vi "Coherent FGV.vi"(7 "Funtion":T1(ring), 8 "error in":errorcluster, 9 "Power(mW)":dbl, 10 "Operating Mode":u16(ring) items=["CW Constant Power", "CW Constant Current", "Pulsed Digital", "Pulsed Analog", "Pulsed Mixed"], 11 "VISA resource name in":refnum<visa-resource-name>) -> (0 "error out":errorcluster, 3 "Laser State":T2)   [LabVIEW 2019, in "Coherent.lvlib"]
uses:
  Coherent.lvlib
  <vilib>/Instr/_visa.llb/VISA Configure Serial Port (Instr).vi
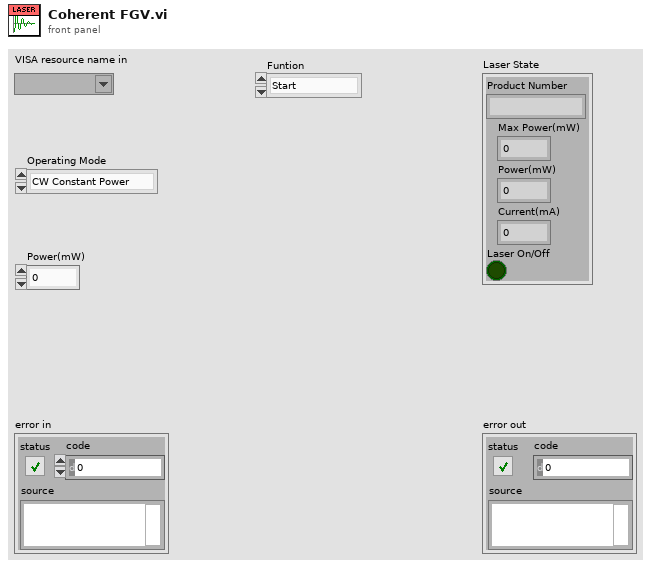
[diagram p1: front panel]
types:
  T1 = enum16{"Start", "Get State", "On", "Off", "Set Power", "Change Mode", "Close"}
  T2 = cluster{"Product Number":string, "Max Power(mW)":dbl, "Power(mW)":dbl, "Current(mA)":dbl, "Laser On/Off":bool}
  T3 = cluster{"Laser State":cluster{"Product Number":string, "Max Power(mW)":dbl, "Power(mW)":dbl, "Current(mA)":dbl, "Laser On/Off":bool}, "VISA resource name":refnum<visa-resource-name>, "Mode":string}
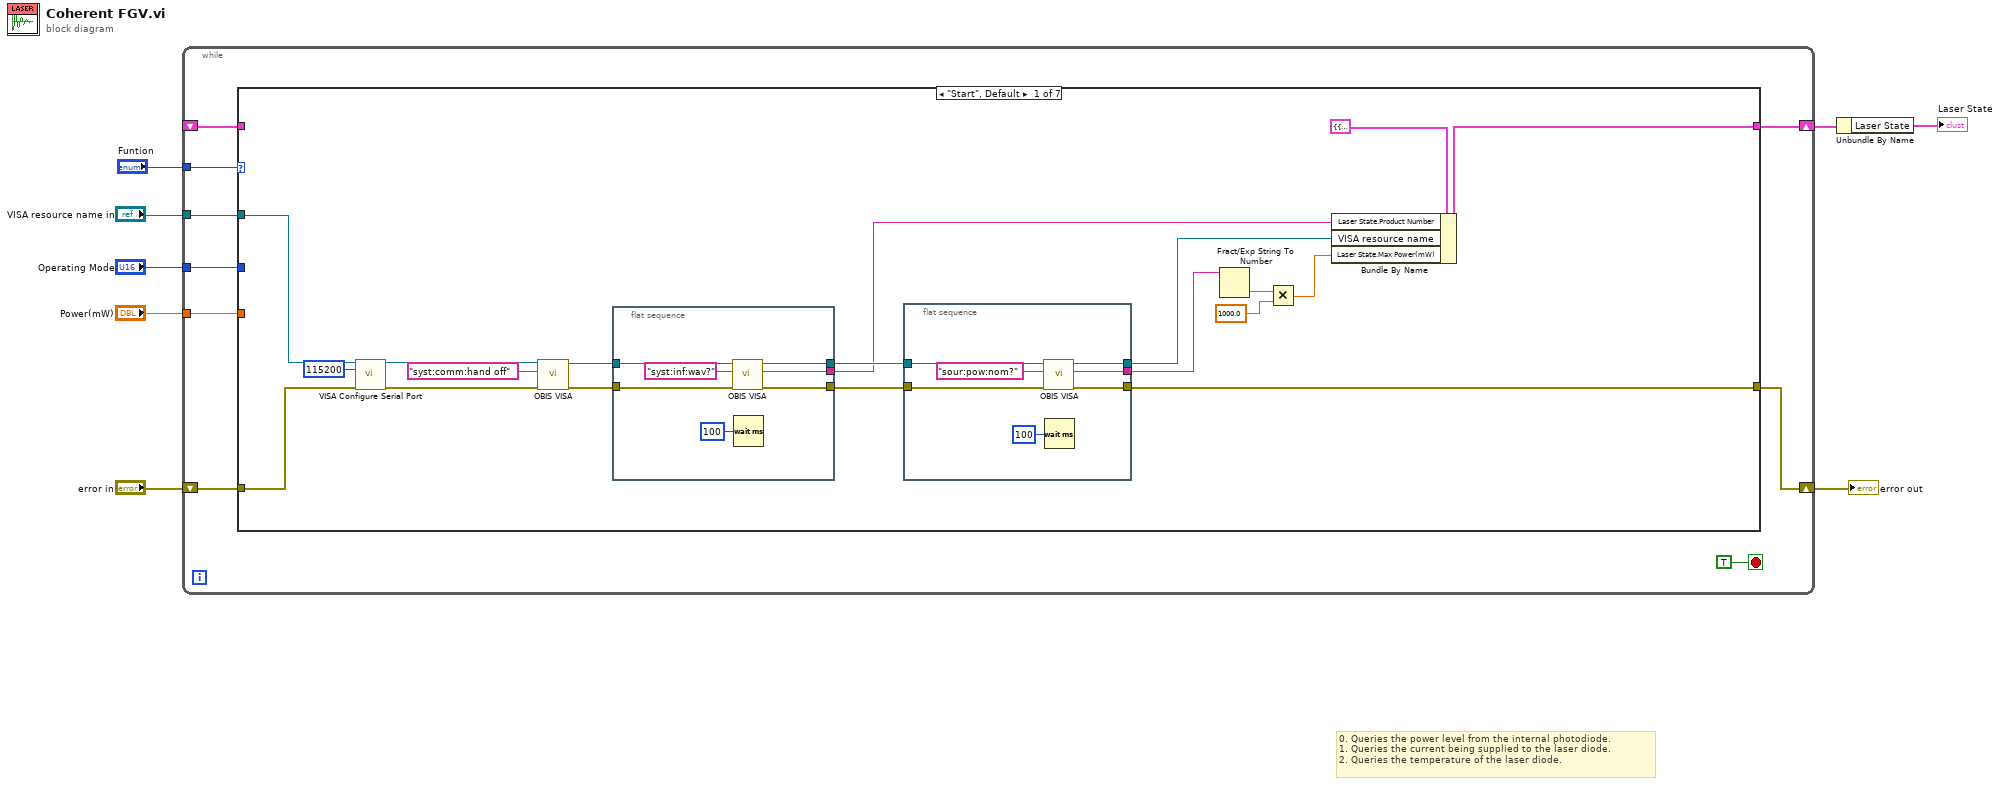
[diagram p0: block diagram]
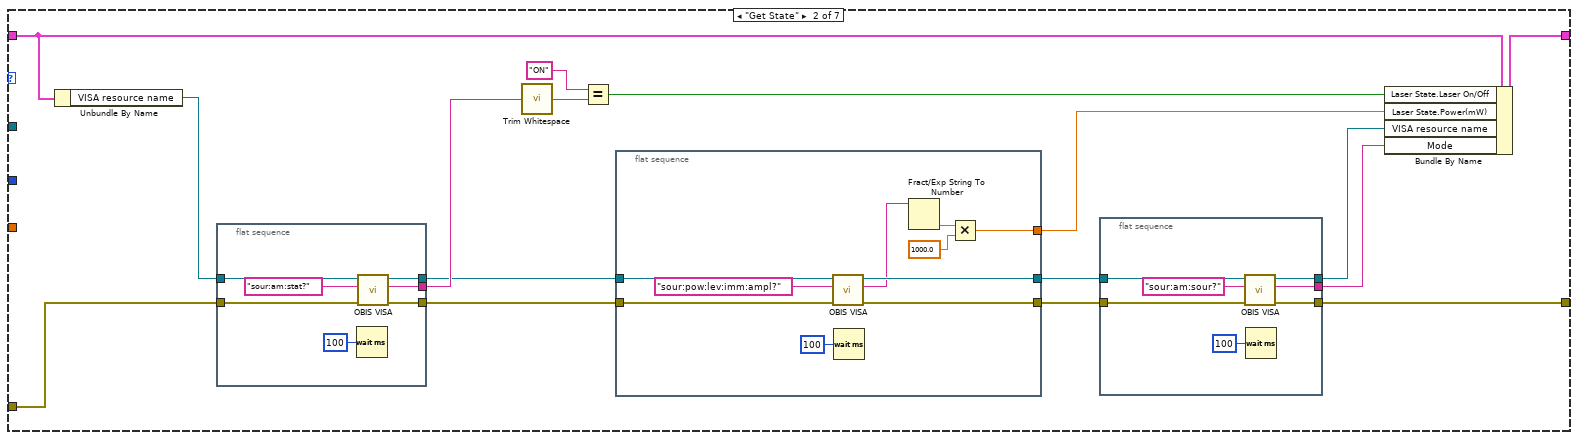
[diagram p2: hidden frame]
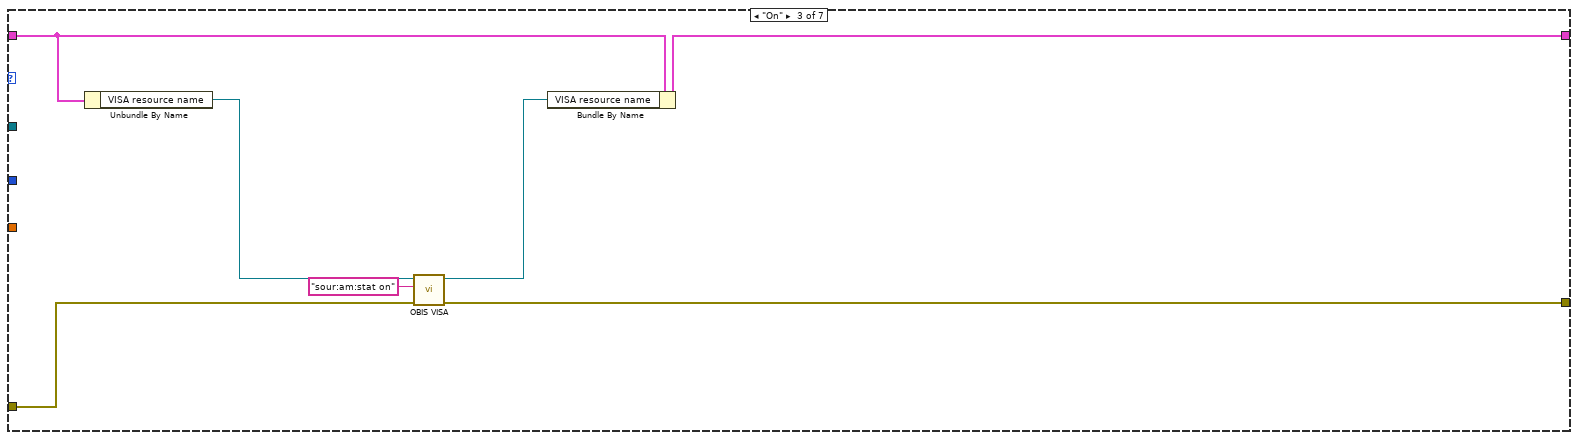
[diagram p3: hidden frame]
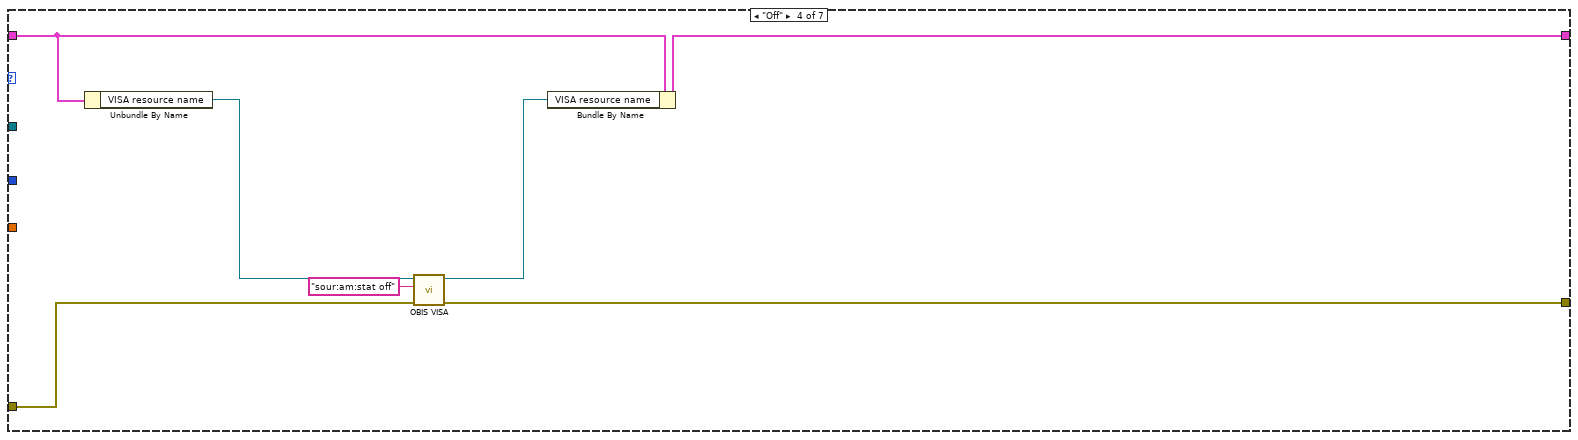
[diagram p4: hidden frame]
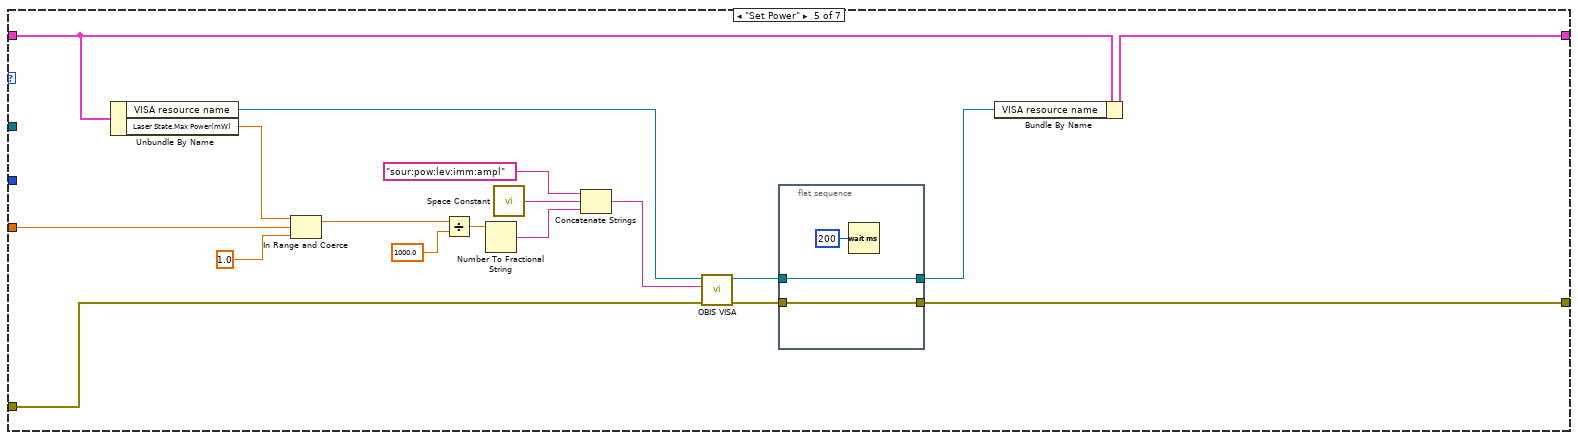
[diagram p5: hidden frame]
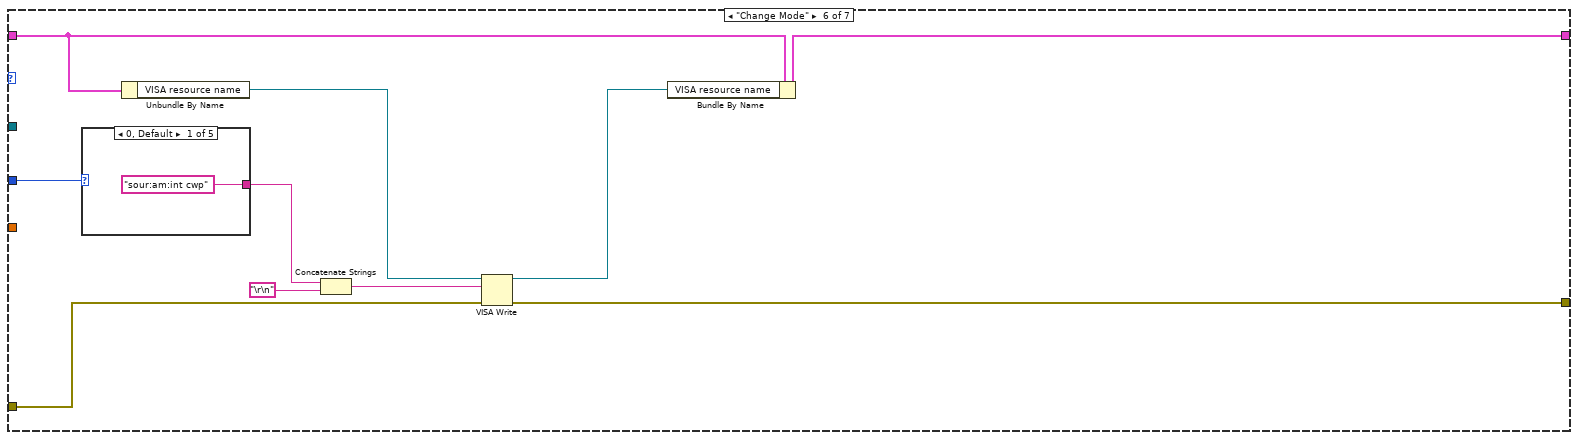
[diagram p6: hidden frame]
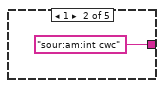
[diagram p7: hidden frame]
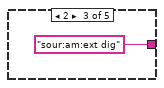
[diagram p8: hidden frame]
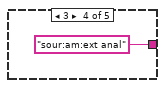
[diagram p9: hidden frame]
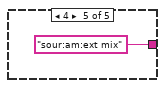
[diagram p10: hidden frame]
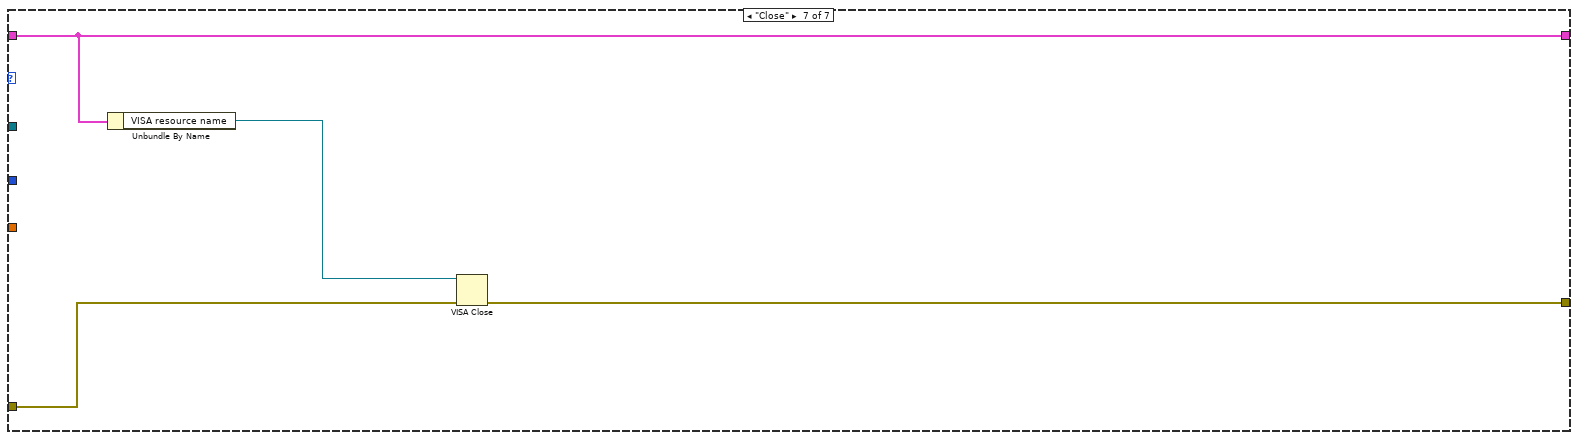
[diagram p11: hidden frame]
diagram:
  # "0. Queries the power level from the internal photodiode.\n1. Queries the current being supplied to the laser diode.\n2. Queries the temperature of the laser diode."
  n1 = while {
    tunnel: "Funtion" -> [w17]
    shift-right: [w14] -> w7
    shift-left: "error in" -> [w16]
    shift-right: [w12] -> w3
    shift-left: _ -> [w13]
    tunnel: "VISA resource name in" -> [w11]
    tunnel: "Operating Mode" -> [w10]
    tunnel: "Power(mW)" -> [w9]
    stop <- TRUE stop-if-true
    n2 = case shown="\"Start\", Default" w17 {
      tunnel: w11 -> [w33 _ _ _ _ _ _]
      tunnel: w16 -> [w32 w65 w96 w103 w122 w131 w144]
      tunnel: [w26 w54 w95 w102 w109 w132 w143] -> w14
      tunnel: w13 -> [_ w63 w94 w101 w113 w129 w142]
      tunnel: [w25 w59 w92 w99 w111 w127 w142] -> w12
      tunnel: w10 -> [_ _ _ _ _ w130 _]
      tunnel: w9 -> [_ _ _ _ w108 _ _]
      frame "Start", Default {
        n3 = call-poly "VISA Configure Serial Port"("VISA resource name"=w33, "baud rate (9600)"=u32 115200, "error in (no error)"=w32) -> ("VISA resource name out"=w35:refnum<visa-resource-name>, "error out"=w31:errorcluster)  [unwired: 11 in]
        n4 = call "OBIS VISA.vi"("error in (no error)"=w31, "write to laser"="syst:comm:hand off", "VISA resource name"=w35) -> ("error out"=w29:errorcluster, "VISA resource name out"=w30:refnum<visa-resource-name>)  [unwired: 6 in, 1 out]
        n5 = flat-sequence {
          tunnel: w30 -> [w43]
          tunnel: w29 -> [w42]
          tunnel: [w41] -> w28
          tunnel: [w40] -> w27
          tunnel: [w37] -> w18
          frame #0 {
            n6 = call "OBIS VISA.vi"("error in (no error)"=w42, "write to laser"="syst:inf:wav?", "VISA resource name"=w43) -> ("error out"=w40:errorcluster, "read from laser"=w37:string, "VISA resource name out"=w41:refnum<visa-resource-name>)  [unwired: 6 in]
            n7 = Wait (ms)(milliseconds to wait=u32 100) -> ()  [unwired: 1 out]
          }
        }
        n8 = flat-sequence {
          tunnel: w28 -> [w50]
          tunnel: w27 -> [w49]
          tunnel: [w48] -> w21
          tunnel: [w47] -> w26
          tunnel: [w44] -> w22
          frame #0 {
            n9 = call "OBIS VISA.vi"("error in (no error)"=w49, "write to laser"="sour:pow:nom?", "VISA resource name"=w50) -> ("error out"=w47:errorcluster, "read from laser"=w44:string, "VISA resource name out"=w48:refnum<visa-resource-name>)  [unwired: 6 in]
            n10 = Wait (ms)(milliseconds to wait=u32 100) -> ()  [unwired: 1 out]
          }
        }
        n11 = Fract/Exp String To Number(string=w22) -> (number=w24:dbl)  [unwired: 3 in, 1 out]
        n12 = Multiply(x=w24, y=1000.0) -> (x*y=w20:dbl)
        n13 = Bundle By Name(cluster=T3 {"Laser State"={"Product Number"="", "Max Power(mW)"=0.0, "Power(mW)"=0.0, "Current(mA)"=0.0, "Laser On/Off"=FALSE}, "VISA resource name"="", "Mode"=""}, "Laser State.Product Number"=w18, "VISA resource name"=w21, "Laser State.Max Power(mW)"=w20) -> (w25:T3)
      }
      frame "Get State" {
        n14 = Unbundle By Name(w63) -> ("VISA resource name"=w62:refnum<visa-resource-name>)
        n15 = flat-sequence {
          tunnel: [w88] -> w66
          tunnel: w65 -> [w87]
          tunnel: [w86] -> w64
          tunnel: w62 -> [w85]
          tunnel: [w84] -> w57
          frame #0 {
            n16 = Wait (ms)(milliseconds to wait=u32 100) -> ()  [unwired: 1 out]
            n17 = call "OBIS VISA.vi"("error in (no error)"=w87, "write to laser"="sour:am:stat?", "VISA resource name"=w85) -> ("error out"=w86:errorcluster, "read from laser"=w88:string, "VISA resource name out"=w84:refnum<visa-resource-name>)  [unwired: 6 in]
          }
        }
        n18 = call <vilib>:"Trim Whitespace.vi"("string"=w66) -> ("trimmed string"=w61:string)  [unwired: 1 in]
        n19 = Equal?(x="ON" ("y"), y=w61) -> (x = y?=w58:bool)
        n20 = flat-sequence {
          tunnel: [w74] -> w56
          tunnel: [w73] -> w55
          tunnel: w57 -> [w75]
          tunnel: w64 -> [w76]
          tunnel: [w67] -> w51
          frame #0 {
            n21 = call "OBIS VISA.vi"("error in (no error)"=w76, "write to laser"="sour:pow:lev:imm:ampl?", "VISA resource name"=w75) -> ("error out"=w73:errorcluster, "read from laser"=w69:string, "VISA resource name out"=w74:refnum<visa-resource-name>)  [unwired: 6 in]
            n22 = Wait (ms)(milliseconds to wait=u32 100) -> ()  [unwired: 1 out]
            n23 = Fract/Exp String To Number(string=w69) -> (number=w71:dbl)  [unwired: 3 in, 1 out]
            n24 = Multiply(x=w71, y=1000.0) -> (x*y=w67:dbl)
          }
        }
        n25 = flat-sequence {
          tunnel: w56 -> [w81]
          tunnel: w55 -> [w80]
          tunnel: [w79] -> w53
          tunnel: [w78] -> w52
          tunnel: [w77] -> w54
          frame #0 {
            n26 = call "OBIS VISA.vi"("error in (no error)"=w80, "write to laser"="sour:am:sour?", "VISA resource name"=w81) -> ("error out"=w77:errorcluster, "read from laser"=w78:string, "VISA resource name out"=w79:refnum<visa-resource-name>)  [unwired: 6 in]
            n27 = Wait (ms)(milliseconds to wait=u32 100) -> ()  [unwired: 1 out]
          }
        }
        n28 = Bundle By Name(cluster=w63, "Laser State.Laser On/Off"=w58, "Laser State.Power(mW)"=w51, "VISA resource name"=w53, "Mode"=w52) -> (w59:T3)
      }
      frame "On" {
        n29 = Unbundle By Name(w94) -> ("VISA resource name"=w93:refnum<visa-resource-name>)
        n30 = call "OBIS VISA.vi"("error in (no error)"=w96, "write to laser"="sour:am:stat on", "VISA resource name"=w93) -> ("error out"=w95:errorcluster, "VISA resource name out"=w91:refnum<visa-resource-name>)  [unwired: 6 in, 1 out]
        n31 = Bundle By Name(cluster=w94, "VISA resource name"=w91) -> (w92:T3)
      }
      frame "Off" {
        n32 = Unbundle By Name(w101) -> ("VISA resource name"=w100:refnum<visa-resource-name>)
        n33 = call "OBIS VISA.vi"("error in (no error)"=w103, "write to laser"="sour:am:stat off", "VISA resource name"=w100) -> ("error out"=w102:errorcluster, "VISA resource name out"=w98:refnum<visa-resource-name>)  [unwired: 6 in, 1 out]
        n34 = Bundle By Name(cluster=w101, "VISA resource name"=w98) -> (w99:T3)
      }
      frame "Set Power" {
        n35 = Unbundle By Name(w113) -> ("VISA resource name"=w112:refnum<visa-resource-name>, "Laser State.Max Power(mW)"=w107:dbl)
        n36 = In Range and Coerce(upper limit=w107, x=w108, lower limit=1.0) -> (coerced(x)=w106:dbl)  [unwired: 1 out]
        n37 = Divide(x=w106, y=1000.0) -> (x/y=w116:dbl)
        n38 = Number To Fractional String(number=w116) -> (F-format string=w119:string)  [unwired: 3 in]
        n39 = call <vilib>:"Space Constant.vi"() -> ("String"=w120:string)
        n40 = Concatenate Strings("sour:pow:lev:imm:ampl", w120, w119) -> (w118:string)
        n41 = call "OBIS VISA.vi"("error in (no error)"=w122, "write to laser"=w118, "VISA resource name"=w112) -> ("error out"=w114:errorcluster, "VISA resource name out"=w115:refnum<visa-resource-name>)  [unwired: 6 in, 1 out]
        n42 = flat-sequence {
          tunnel: [w124] -> w110
          tunnel: w115 -> [w124]
          tunnel: [w123] -> w109
          tunnel: w114 -> [w123]
          frame #0 {
            n43 = Wait (ms)(milliseconds to wait=u32 200) -> ()  [unwired: 1 out]
          }
        }
        n44 = Bundle By Name(cluster=w113, "VISA resource name"=w110) -> (w111:T3)
      }
      frame "Change Mode" {
        n45 = case shown="0, Default" w130 {
          tunnel: ["sour:am:int cwp" "sour:am:int cwc" "sour:am:ext dig" "sour:am:ext anal" "sour:am:ext mix"] -> w135
          frame 0, Default {
          }
          frame 1 {
          }
          frame 2 {
          }
          frame 3 {
          }
          frame 4 {
          }
        }
        n46 = Unbundle By Name(w129) -> ("VISA resource name"=w128:refnum<visa-resource-name>)
        n47 = Concatenate Strings(w135, "\r\n") -> (w134:string)
        n48 = VISA Write(VISA resource name=w128, write buffer=w134, error in (no error)=w131) -> (VISA resource name out=w126:refnum<visa-resource-name>, error out=w132:errorcluster)  [unwired: 1 out]
        n49 = Bundle By Name(cluster=w129, "VISA resource name"=w126) -> (w127:T3)
      }
      frame "Close" {
        n50 = Unbundle By Name(w142) -> ("VISA resource name"=w141:refnum<visa-resource-name>)
        n51 = VISA Close(VISA resource name=w141, error in (no error)=w144) -> (error out=w143:errorcluster)
      }
    }
  }
  "error out" <- w7
  n52 = Unbundle By Name(w3) -> ("Laser State"=→"Laser State":T2)
